vi "TB-Init Logging.vi"(0 "state in":T5, 1 "Slack":T4, 2 "Params":T1={"Low cutoff (kHz)"=0.0, "High cutoff (kHz)"=0.0, "Duration (min)"=0.0, "dB SPL"=0.0, "Waveform"=enum."Noise", "WAVfile"=path "", "refWav"=path "", "use mic correction"=FALSE, "micCorrFile"=path "", "Pistonphone Level (dB SPL)"=0.0, "Sampling rate (Hz)"=0.0, "Buffer length (s)"=0.0, "Stream mic"=FALSE, "Fine adjust"={"Max"=0.0, "Min"=0.0}, "Mic gain"=0.0, "atten"=0.0, "Allow Slack"=FALSE, "max starts"=0, "Freq (kHz)"=8.0, "Tma (s)"=0.0, "Streamed"=[], "Drive"="", "Speaker"="", "Mic"="", "Analysis"={"Method"=enum."Default", "resol (Hz)"=0.0, "nfreq"=0, "signal"=""}, "exposeAtten"=0.0, "Digital"=""}, 7 "Level":dbl, 11 "error in (no error)":errorcluster, 13 "Pistonphone factor":dbl) -> (3 "Log":T3, 4 "state out":T5, 15 "error out":errorcluster)   [LabVIEW 2020]
uses:
  Typedefs/TB-Runtime state.ctl
  <vilib>/sound2/lvsound2.llb/Sound File Refnum.ctl
  Typedefs/TB-Setup Log.ctl
  Typedefs/TB-Analysis State.ctl
  Typedefs/TB-Slack State.ctl
  Typedefs/TB-Log.ctl
  Typedefs/TB-Parameters.ctl
  Typedefs/TB-Analysis Parameters.ctl
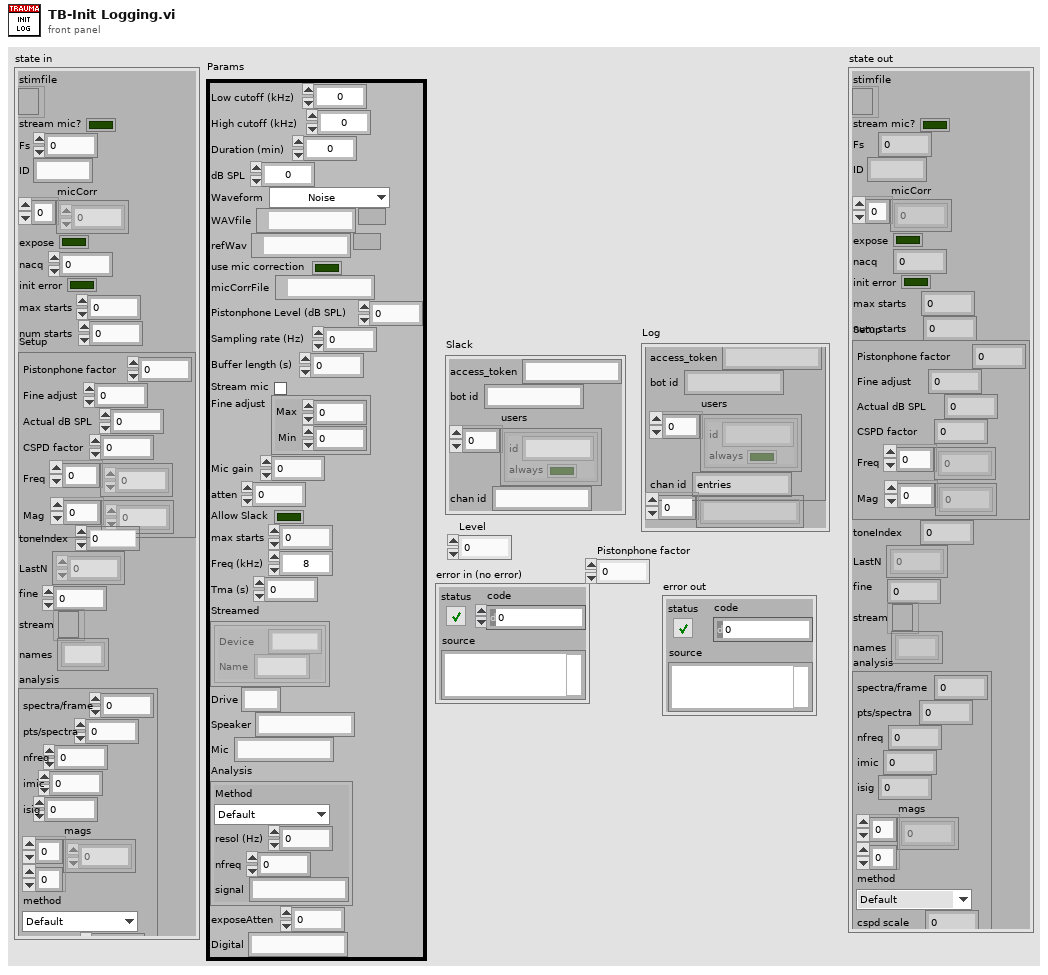
[diagram p1: front panel]
types:
  T1 = typedef "TB-Parameters.ctl" = cluster{"Low cutoff (kHz)":dbl, "High cutoff (kHz)":dbl, "Duration (min)":dbl, "dB SPL":dbl, "Waveform":enum16{"Noise", "File", "Tone"}, "WAVfile":path, "refWav":path, "use mic correction":bool, "micCorrFile":path, "Pistonphone Level (dB SPL)":dbl, "Sampling rate (Hz)":dbl, "Buffer length (s)":dbl, "Stream mic":bool, "Fine adjust":cluster{"Max":dbl, "Min":dbl}, "Mic gain":dbl, "atten":dbl, "Allow Slack":bool, "max starts":i32, "Freq (kHz)":dbl, "Tma (s)":dbl, "Streamed":cluster{"Device":string, "Name":string}[], "Drive":string, "Speaker":string, "Mic":string, "Analysis":T2, "exposeAtten":dbl, "Digital":string}
  T2 = typedef "TB-Analysis Parameters.ctl" = cluster{"Method":enum16{"Default", "Periodogram", "Cross-spectrum"}, "resol (Hz)":dbl, "nfreq":i32, "signal":string}
  T3 = typedef "TB-Log.ctl" = cluster{"Slack":T4, "entries":string[]}
  T4 = typedef "TB-Slack State.ctl" = cluster{"access_token":string, "bot id":string, "users":cluster{"id":string, "always":bool}[], "chan id":string}
  T5 = typedef "TB-Runtime state.ctl" = cluster{"stimfile":T6, "stream mic?":bool, "Fs":dbl, "ID":string, "micCorr":dbl[], "expose":bool, "nacq":i32, "init error":bool, "max starts":i32, "num starts":i32, "Setup":T7, "toneIndex":i32, "LastN":dbl[], "fine":dbl, "stream":refnum<file>, "names":string[], "analysis":T8}
  T6 = typedef "Sound File Refnum.ctl" = refnum<file>
  T7 = typedef "TB-Setup Log.ctl" = cluster{"Pistonphone factor":dbl, "Fine adjust":dbl, "Actual dB SPL":dbl, "CSPD factor":dbl, "Freq":dbl[], "Mag":dbl[]}
  T8 = typedef "TB-Analysis State.ctl" = cluster{"spectra/frame":i32, "pts/spectra":i32, "nfreq":i32, "imic":i32, "isig":i32, "mags":dbl[][], "method":enum16{"Default", "Periodogram", "Cross-spectrum"}, "cspd scale":dbl}
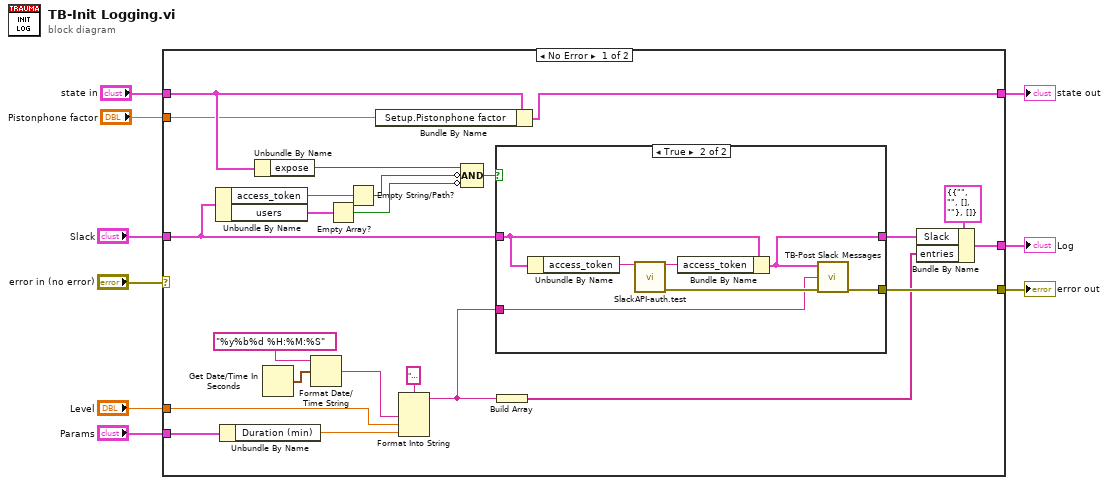
[diagram p0: block diagram]
diagram:
  n1 = case shown="No Error" "error in (no error)" {
    selector: "error in (no error)" -> [_ w41]
    tunnel: "Slack" -> [w28 _]
    tunnel: [w25 _] -> w8
    tunnel: [w24 w41] -> w6
    tunnel: "state in" -> [w12 w40]
    tunnel: "Params" -> [w21 _]
    tunnel: "Level" -> [w16 _]
    tunnel: "Pistonphone factor" -> [w11 _]
    tunnel: [w10 w40] -> w1
    frame No Error {
      n2 = Unbundle By Name(w28) -> ("access_token"=w32:string, "users"=w31:cluster{"id":string, "always":bool}[])
      n3 = Unbundle By Name(w21) -> ("Duration (min)"=w15:dbl)
      n4 = Unbundle By Name(w12) -> ("expose"=w23:bool)
      n5 = Get Date/Time In Seconds() -> (seconds since 1Jan1904=w20:timestamp)
      n6 = Format Date/Time String(time format string (%c)="%y%b%d %H:%M:%S", seconds (now)=w20) -> (date/time string=w17:string)  [unwired: 1 in]
      n7 = Empty Array?(array=w31) -> (empty?=w29:bool)
      n8 = Empty String/Path?(string/path=w32) -> (empty?=w30:bool)
      n9 = Bundle By Name(cluster=w12, "Setup.Pistonphone factor"=w11) -> (w10:T5)
      n10 = Format Into String(format string="Exposure started %s\n%.1f dB SPL for %#g minutes\n", w17, w16, w15) -> (resulting string=w13:string)  [unwired: 2 in, 1 out]
      n11 = Compound Arithmetic op=AND(w23, invert w30, invert w29) -> (w22:bool)
      n12 = case shown="True" w22 {
        tunnel: w28 -> [_ w36]
        tunnel: [_ w35] -> w26
        tunnel: [_ w39] -> w24
        tunnel: w13 -> [_ w33]
        frame False {
        }
        frame True {
          n13 = Unbundle By Name(w36) -> ("access_token"=w37:string)
          n14 = call "SlackAPI-auth.test.vi"("token"=w37) -> ("token out"=w34:string, "error out"=w38:errorcluster)  [unwired: 13 in]
          n15 = Bundle By Name(cluster=w36, "access_token"=w34) -> (w35:T4)
          n16 = call "TB-Post Slack Messages.vi"("Slack"=w35, "Message"=w33, "error in (no error)"=w38) -> ("error out"=w39:errorcluster)  [unwired: 12 in]
        }
      }
      n17 = Build Array(w13) -> (w14:string[])
      n18 = Bundle By Name(cluster=T3 {"Slack"={"access_token"="", "bot id"="", "users"=[], "chan id"=""}, "entries"=[]} ("Log"), "Slack"=w26, "entries"=w14) -> (w25:T3)
    }
    frame Error {
    }
  }
  "error out" <- w6
  "state out" <- w1
  "Log" <- w8
